vi "reconnect.vi"(8 "error in (no error)":errorcluster, 11 "AlCS in":refnum<class "AlCS.lvclass">) -> (0 "error out":errorcluster, 3 "AlCS out":refnum<class "AlCS.lvclass">)   [LabVIEW 2016, in "AlCS.lvclass"]
uses:
  AlCS.lvclass
  AlCS.lvclass/AlCS.ctl
  ts_labview_tcp/TCPClient/TCPClient.lvclass
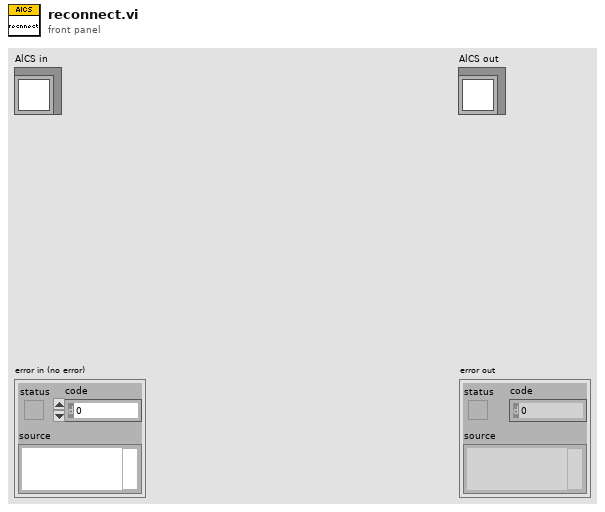
[diagram p1: front panel]
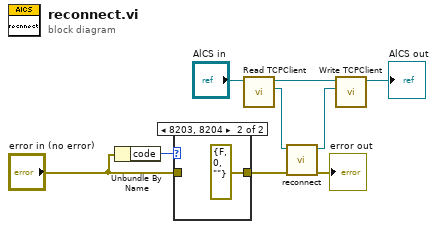
[diagram p0: block diagram]
diagram:
  n1 = Unbundle By Name("error in (no error)") -> ("code"=w9:i32)
  n2 = case shown="8203, 8204" w9 {
    tunnel: [w10 errorcluster {"status"=FALSE, "code"=0, "source"=""} ("error in (no error)")] -> w2
    tunnel: "error in (no error)" -> [w10 _]
    frame 0, Default {
    }
    frame 8203, 8204 {
    }
  }
  n3 = call "Read TCPClient.vi"("AlCS in"="AlCS in") -> ("TCPClient.lvclass"=w3:refnum<class "TCPClient.lvclass">, "AlCS out"=w7:refnum<class "AlCS.lvclass">)  [unwired: 8 in, 1 out]
  n4 = call-dynamic "reconnect.vi"("error in (no error)"=w2, "TCPCommunicator in"=w3) -> ("error out"=→"error out":errorcluster, "TCPCommunicator out"=w4:refnum<class "TCPClient.lvclass">)  [unwired: 8 in]
  n5 = call "Write TCPClient.vi"("TCPClient.lvclass"=w4, "AlCS in"=w7) -> ("AlCS out"=→"AlCS out":refnum<class "AlCS.lvclass">)  [unwired: 8 in, 1 out]
